vi "Assign Value.vi"(8 "error in (no error)":errorcluster, 10 "Assigned Value":refnum<class "Abs_Value.lvclass">, 11 "Abs_U32 Integer in":refnum<class "Abs_U32 Integer.lvclass">) -> (0 "error out":errorcluster, 3 "Abs_U32 Integer out":refnum<class "Abs_U32 Integer.lvclass">)   [LabVIEW 2021, in "Abs_U32 Integer.lvclass"]
uses:
  Abs_U32 Integer.lvclass
  Value/Abs_Value.lvclass
  Numeric/Abs_Numeric.lvclass
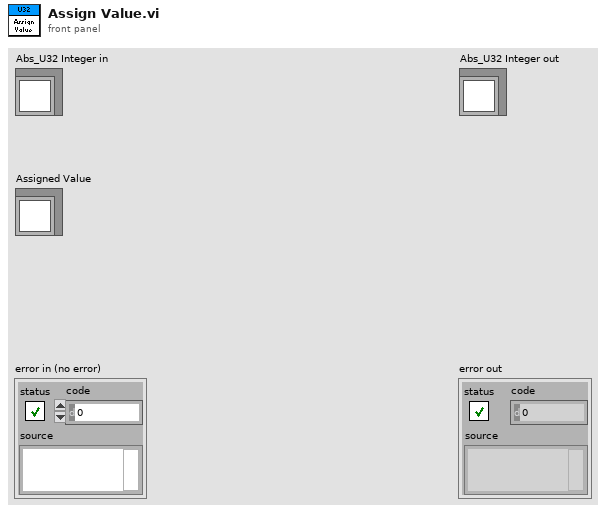
[diagram p1: front panel]
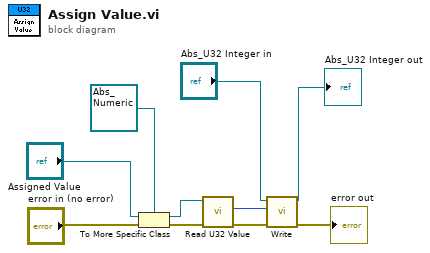
[diagram p0: block diagram]
diagram:
  n1 = To More Specific Class(target class=refnum<class "Abs_Numeric.lvclass"> refnum ("Abs_Numeric.lvclass"), reference="Assigned Value", error in="error in (no error)") -> (specific class reference=w6:refnum<class "Abs_Numeric.lvclass">, error out=w7:errorcluster)
  n2 = call-dynamic "Read U32 Value.vi"("error in (no error)"=w7, "Numeric in"=w6) -> ("error out"=w5:errorcluster, "U32"=w4:u32)  [unwired: 7 in, 1 out]
  n3 = call-dynamic "Write.vi"("error in (no error)"=w5, "Value"=w4, "Double Float.lvclass_340760 in"="Abs_U32 Integer in") -> ("error out"=→"error out":errorcluster, "Double Float.lvclass_340760 out"=→"Abs_U32 Integer out":refnum<class "Abs_U32 Integer.lvclass">)  [unwired: 7 in]
